vi "PMJD T027 SubVI05.vi"(0 "P":dbl, 1 "XC":dbl, 2 "f":dbl[][](array[numeric]), 3 "Q":dbl, 4 "YC":dbl) -> (5 "upq":dbl)   [LabVIEW 2020]
doc: "PINEDA MENDEZ JOB DANIEL 4MV6 SVA 2022/1\nT027 SubVI05\nEste subvi calcula los momentos centrales(upq) dados los parametros P, Q, Xc, Yc y f."
panel:
  # "PINEDA MENDEZ JOB DANIEL    4MV6    SVA    2022/1\nT027     SubVI05    Calculo de momentos centrales upq"
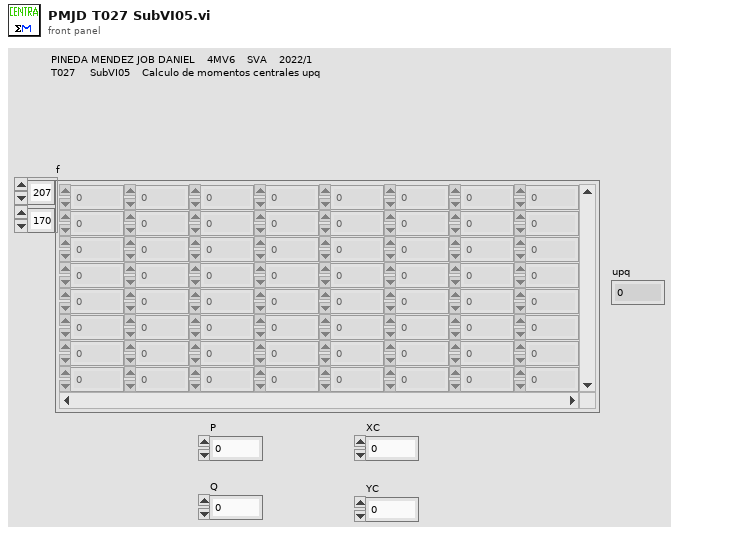
[diagram p1: front panel]
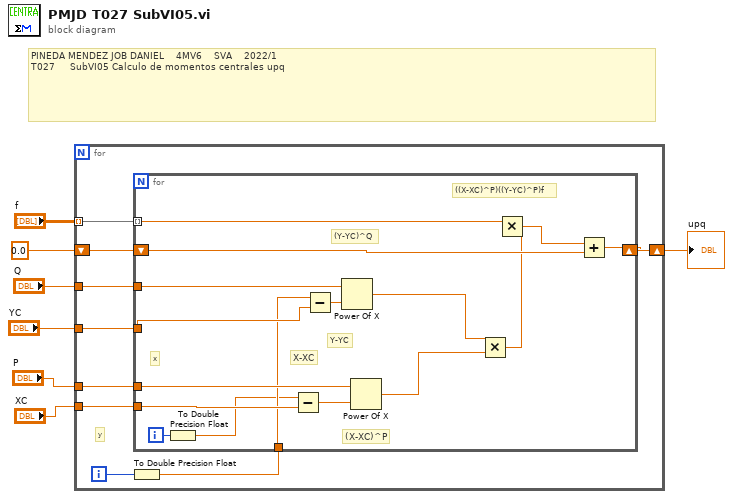
[diagram p0: block diagram]
diagram:
  # "PINEDA MENDEZ JOB DANIEL    4MV6    SVA    2022/1\nT027     SubVI05 Calculo de momentos centrales upq"
  n1 = for {
    tunnel: "f" -> [w16] mode=indexing
    tunnel: "P" -> [w15]
    tunnel: "Q" -> [w14]
    shift-right: [w13] -> w3
    shift-left: 0.0 -> [w12]
    tunnel: "XC" -> [w11]
    tunnel: "YC" -> [w10]
    i -> [w9]
    # "y"
    n2 = To Double Precision Float(number=w9) -> (double precision float=w8:dbl)
    n3 = for {
      tunnel: w16 -> [w20] mode=indexing
      tunnel: w15 -> [w32]
      tunnel: w14 -> [w30]
      shift-right: [w28] -> w13
      shift-left: w12 -> [w27]
      tunnel: w11 -> [w25]
      tunnel: w10 -> [w23]
      tunnel: w8 -> [w18]
      i -> [w31]
      # "Y-YC"
      # "X-XC"
      # "((X-XC)^P)((Y-YC)^P)f"
      # "(Y-YC)^Q"
      # "(X-XC)^P"
      # "x"
      n4 = To Double Precision Float(number=w31) -> (double precision float=w17:dbl)
      n5 = Subtract(x=w17, y=w25) -> (x-y=w26:dbl)
      n6 = Subtract(x=w18, y=w23) -> (x-y=w24:dbl)
      n7 = Power Of X(1:w24, 2:w30) -> (0:w22:dbl)
      n8 = Power Of X(1:w26, 2:w32) -> (0:w21:dbl)
      n9 = Multiply(x=w22, y=w21) -> (x*y=w19:dbl)
      n10 = Multiply(x=w20, y=w19) -> (x*y=w29:dbl)
      n11 = Add(x=w29, y=w27) -> (x+y=w28:dbl)
    }
  }
  "upq" <- w3
